vi "Read Record.vi"(8 "error in (no error)":errorcluster, 10 "Keypad Screen":dbl, 11 "Configuration Database in":refnum<class "Configuration Database.lvclass">) -> (0 "error out":errorcluster, 3 "Configuration Database out":refnum<class "Configuration Database.lvclass">)   [LabVIEW 2019, in "Configuration Database.lvlib" / "Configuration Database.lvclass"]
uses:
  Configuration Database.lvclass
  <vilib>/ActorFramework/Actor/Actor.lvclass
  ATM Controller/ATM Controller Messages/Get DB Record Msg/Get DB Record Msg.lvclass
  ATM Controller/ATM Controller Messages/Set State Msg/Set State Msg.lvclass
  ATM Controller/ATM Controller/State -Enum.ctl
  ATM Controller/ATM Controller/ATM Controller.lvclass
  ATM Controller/ATM Controller Messages/Set Message Msg/Set Message Msg.lvclass
  Sim Display Console Actor/ATM Controller/Message Name.ctl
  Sim Display Console Actor/ATM Controller/Sim Display Console Actor.lvclass
  C:/Program Files (x86)/National Instruments/LabVIEW 2019/vi.lib/ActorFramework/Actor/Actor.lvclass
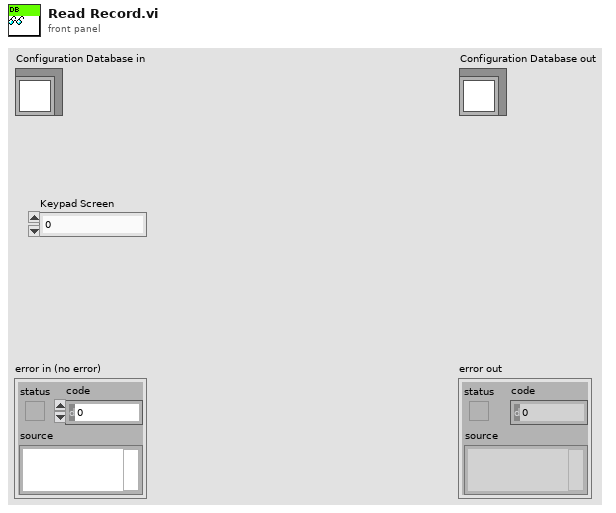
[diagram p1: front panel]
types:
  T1 = typedef "Sim Display Console Actor.lvlib/Sim Display Console Actor.lvclass/Message Name.ctl" = enum16{"Welcome", "Login", "Idle", "Invalid Login", "Terminate Session", "Deposit", "Withdrawal", "Fast Cash $50", "Withdrawal Complete", "Withdrawal Failed", "Balance Inquiry"}
  T2 = typedef "ATM Controller.lvlib/ATM Controller.lvclass/State -Enum.ctl" = enum16{"Initial", "Idle", "Login", "Balance Inquiry", "Deposit", "Withdrawal", "Fast Cash", "Terminate", "Inactivity Timeout"}
  T3 = typedef "Configuration Database.lvlib/Configuration Database.lvclass/Record -Cluster.ctl" = cluster{"First name":string, "Last Name":string, "Account Number":u16, "Balance":u32}
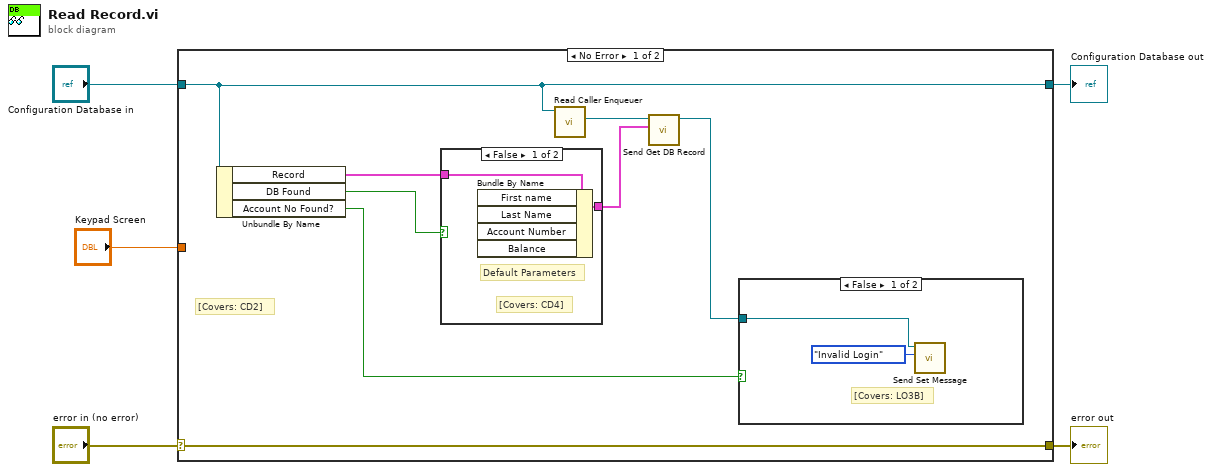
[diagram p0: block diagram]
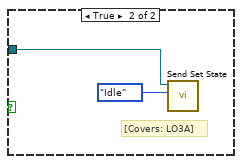
[diagram p2: hidden frame]
diagram:
  n1 = case shown="No Error" "error in (no error)" {
    selector: "error in (no error)" -> [w13 w21]
    tunnel: [w13 w21] -> w4
    tunnel: [w12 w22] -> w2
    tunnel: "Configuration Database in" -> [w12 w22]
    tunnel: "Keypad Screen" -> [_ _]
    frame No Error {
      # "[Covers: CD2]"
      n2 = Unbundle By Name(w12) -> ("Record"=w10:T3, "DB Found"=w8:bool, "Account No Found?"=w7:bool)
      n3 = case shown="False" w8 {
        tunnel: w10 -> [w19 w20]
        tunnel: [w18 w20] -> w9
        frame False {
          # "[Covers: CD4]"
          # "Default Parameters"
          n4 = Bundle By Name(cluster=w19) -> (w18:T3)  [unwired: 4 in]
        }
        frame True {
        }
      }
      n5 = call <vilib>:"Read Caller Enqueuer.vi"("Actor"=w12) -> ("Caller Enqueuer"=w11:refnum<class "Message Enqueuer.lvclass">)  [unwired: 10 in]
      n6 = call "Send Get DB Record.vi"("Record"=w9, "Message Enqueuer"=w11) -> ("Message Enqueuer out"=w6:refnum<class "Message Enqueuer.lvclass">)  [unwired: 8 in, 1 out]
      n7 = case shown="False" w7 {
        tunnel: w6 -> [w15 w16]
        frame False {
          # "[Covers: LO3B]"
          n8 = call "Send Set Message.vi"("Message Name"=Message_Name."Invalid Login", "Message Enqueuer"=w15) -> ()  [unwired: 8 in, 2 out]
        }
        frame True {
          # "[Covers: LO3A]"
          n9 = call "Send Set State.vi"("State"=State_-Enum."Idle", "Message Enqueuer"=w16) -> ()  [unwired: 8 in, 2 out]
        }
      }
    }
    frame Error {
    }
  }
  "error out" <- w4
  "Configuration Database out" <- w2
